vi "Teleop.vi"(10 "Match Info":T1={"Autonomous Elapsed Seconds"=0.0, "TeleOp Elapsed Seconds"=0.0, "Disabled Elapsed Seconds"=0.0, "Visited Autonomous"=FALSE, "Visited TeleOp"=FALSE, "Visited Disabled"=FALSE, "Autonomous Settings"={"Autonomous Style"=enum."Independent", "VI Refnum"=refnum}}, 11 "Call Context":T2) -> ()   [LabVIEW 2019]
doc: "This VI is called for each enabled TeleOp packet received from the DS. It is typically used to read from joysticks and other inputs and update I/O or setpoints for timed control loops. It should complete and return within 20 milliseconds or risk missing DS packets."
uses:
  <vilib>/Rock Robotics/WPI/DriverStation/WPI_DriverStationDerivedRobotMode.ctl
  <vilib>/Rock Robotics/WPI/DriverStation/WPI_DriverStationMatch Info.ctl
  Framework/Robot Global Data.vi
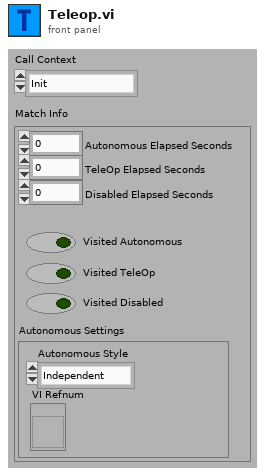
[diagram p1: front panel]
types:
  T1 = typedef "WPI_DriverStationMatch Info.ctl" = cluster{"Autonomous Elapsed Seconds":dbl, "TeleOp Elapsed Seconds":dbl, "Disabled Elapsed Seconds":dbl, "Visited Autonomous":bool, "Visited TeleOp":bool, "Visited Disabled":bool, "Autonomous Settings":cluster{"Autonomous Style":enum16{"Iterative", "Independent"}, "VI Refnum":refnum<vi>}}
  T2 = typedef "WPI_DriverStationDerivedRobotMode.ctl" = enum16{"Init", "Execute", "Stop"}
  T3 = typedef "Command Status Info.ctl" = cluster{"Name":string, "Status":T4, "notifier out":T5}
  T4 = typedef "Completion Status.ctl" = enum16{"Successful", "Aborted", "Incomplete"}
  T5 = typedef "Completion Notifier.ctl" = refnum<notifier>
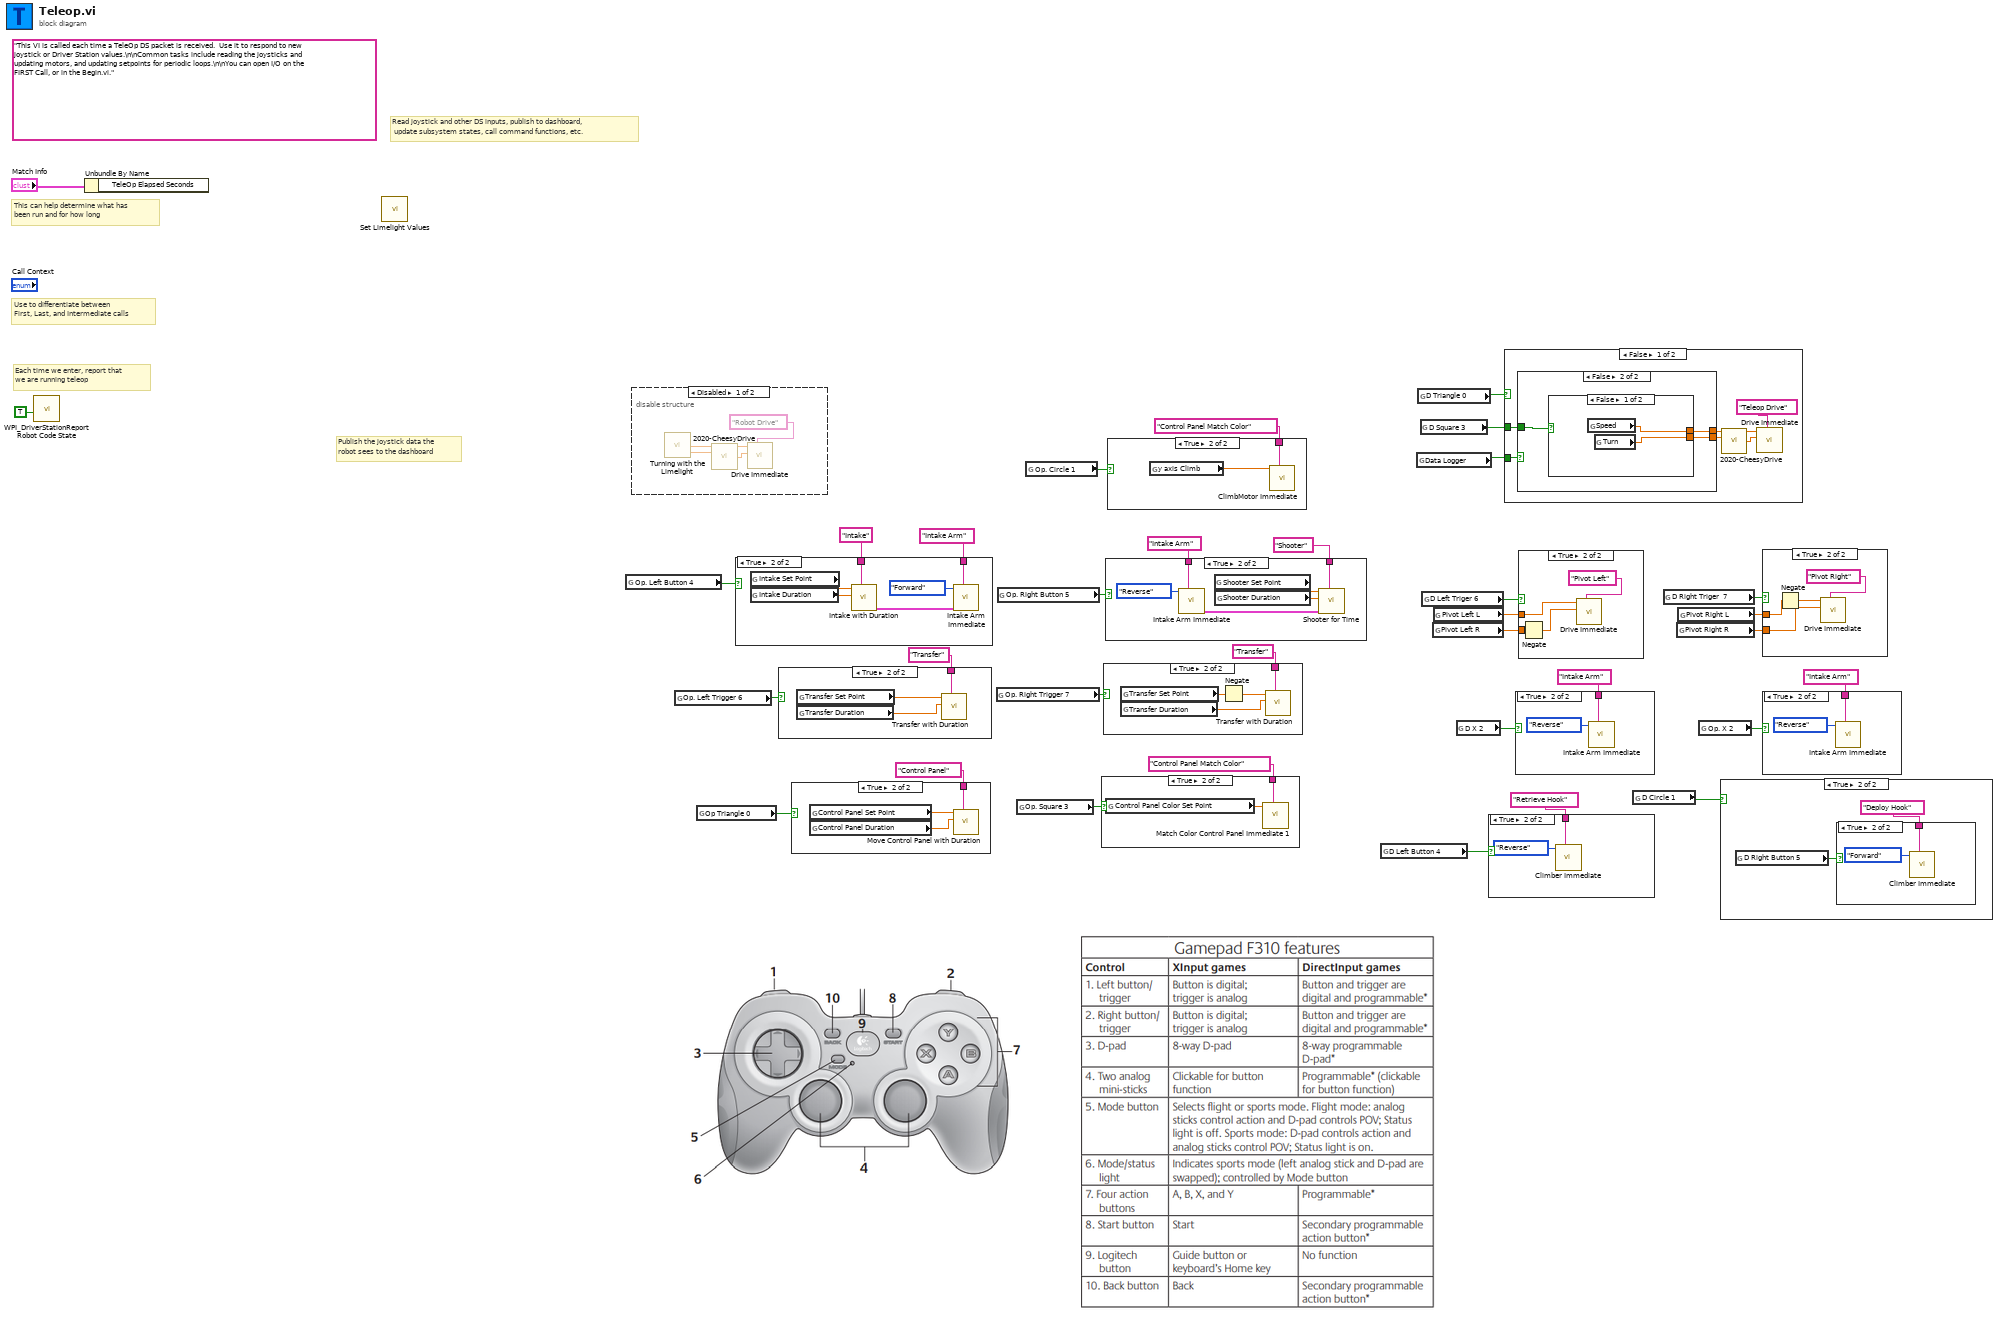
[diagram p0: block diagram]
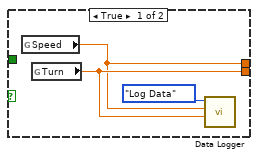
[diagram p8: hidden frame]
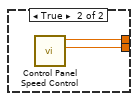
[diagram p9: hidden frame]
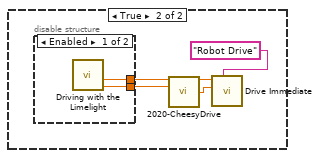
[diagram p10: hidden frame]
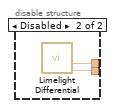
[diagram p11: hidden frame]
diagram:
  (unwired) "This VI is called each time a TeleOp DS packet is received.  Use it to respond to new joystick or Driver Station values.\n\nCommon tasks include reading the joysticks and updating motors, and updating setpoints for periodic loops.\n\nYou can open I/O on the FIRST Call, or in the Begin.vi."
  # "Publish the joystick data the\nrobot sees to the dashboard"
  # "Read joystick and other DS inputs, publish to dashboard,\n update subsystem states, call command functions, etc."
  # "Each time we enter, report that\nwe are running teleop"
  # "Use to differentiate between\nFirst, Last, and Intermediate calls"
  # "This can help determine what has\nbeen run and for how long"
  n1 = call <vilib>:"WPI_DriverStationReport Robot Code State.vi"("TeleOp"=TRUE ("Autonomous")) -> ()  [unwired: 10 in, 1 out]
  n2 = Unbundle By Name("Match Info") -> ()  [unwired: 1 out]
  n3 = call "Set Limelight Values.vi"() -> ()  [unwired: 12 in]
  n4 = global read "Robot Global Data.vi" "Op. Left Button 4"() -> (w32:bool)
  n5 = disable-structure shown="Disabled" {
    frame Disabled {
      n6 = call "Turning with the Limelight.vi"() -> ("TurnCommand"=w38:dbl, "Speed Command"=w39:dbl)  [unwired: 9 in, 1 out]
      n7 = call "2020-CheesyDrive.vi"("Throttle"=w39, "Wheel"=w38) -> ("Left PWM"=w37:dbl, "Right PWM"=w36:dbl)  [unwired: 12 in]
      n8 = call "Drive Immediate.vi"("Description"="Robot Drive", "Right Setpoint"=w36, "Left Setpoint"=w37) -> ()  [unwired: 8 in, 1 out]
    }
    frame Enabled {
    }
  }
  n9 = global read "Robot Global Data.vi" "Op. Left Trigger 6"() -> (w26:bool)
  n10 = global read "Robot Global Data.vi" "Op Triangle 0"() -> (w19:bool)
  n11 = case shown="True" w32 {
    tunnel: "Intake" ("refnum name") -> [_ w45]
    tunnel: "Intake Arm" ("refnum name") -> [_ w41]
    frame False {
    }
    frame True {
      n12 = global read "Robot Global Data.vi" "Intake Set Point"() -> (w44:dbl)
      n13 = global read "Robot Global Data.vi" "Intake Duration"() -> (w43:dbl)
      n14 = call "Intake with Duration.vi"("Description"=w45, "Duration (s)"=w43, "Setpoint"=w44) -> ("Command Info Out"=w40:T3)  [unwired: 8 in]
      n15 = call "Intake Arm Immediate.vi"("Description"=w41, "Command Info In"=w40, "Relay Value"=enum16{"Off", "On", "Forward", "Reverse"}."Forward") -> ()  [unwired: 8 in, 1 out]
    }
  }
  n16 = case shown="True" w26 {
    tunnel: "Transfer" ("refnum name") -> [_ w48]
    frame False {
    }
    frame True {
      n17 = global read "Robot Global Data.vi" "Transfer Set Point"() -> (w47:dbl)
      n18 = global read "Robot Global Data.vi" "Transfer Duration"() -> (w46:dbl)
      n19 = call "Transfer with Duration.vi"("Description"=w48, "Duration (s)"=w46, "Setpoint"=w47) -> ()  [unwired: 8 in, 1 out]
    }
  }
  n20 = case shown="True" w19 {
    tunnel: "Control Panel" ("refnum name") -> [_ w51]
    frame False {
    }
    frame True {
      n21 = global read "Robot Global Data.vi" "Control Panel Set Point"() -> (w50:dbl)
      n22 = global read "Robot Global Data.vi" "Control Panel Duration"() -> (w49:dbl)
      n23 = call "Move Control Panel with Duration.vi"("Description"=w51, "Duration (s)"=w49, "Setpoint"=w50) -> ()  [unwired: 8 in, 1 out]
    }
  }
  n24 = global read "Robot Global Data.vi" "Op. Right Trigger 7"() -> (w27:bool)
  n25 = global read "Robot Global Data.vi" "Op. Right Button 5"() -> (w28:bool)
  n26 = global read "Robot Global Data.vi" "Op. Square 3"() -> (w16:bool)
  n27 = global read "Robot Global Data.vi" "Op. Circle 1"() -> (w4:bool)
  n28 = case shown="True" w16 {
    tunnel: "Control Panel Match Color" ("refnum name") -> [_ w53]
    frame False {
    }
    frame True {
      n29 = global read "Robot Global Data.vi" "Control Panel Color Set Point"() -> (w52:dbl)
      n30 = call "Match Color Control Panel Immediate 1.vi"("Description"=w53, "Setpoint"=w52) -> ()  [unwired: 9 in, 1 out]
    }
  }
  n31 = case shown="True" w27 {
    tunnel: "Transfer" ("refnum name") -> [_ w57]
    frame False {
    }
    frame True {
      n32 = global read "Robot Global Data.vi" "Transfer Set Point"() -> (w55:dbl)
      n33 = global read "Robot Global Data.vi" "Transfer Duration"() -> (w54:dbl)
      n34 = Negate(x=w55) -> (-x=w56:dbl)
      n35 = call "Transfer with Duration.vi"("Description"=w57, "Duration (s)"=w54, "Setpoint"=w56) -> ()  [unwired: 8 in, 1 out]
    }
  }
  n36 = case shown="True" w28 {
    tunnel: "Shooter" ("refnum name") -> [_ w63]
    tunnel: "Intake Arm" ("refnum name") -> [_ w58]
    frame False {
    }
    frame True {
      n37 = call "Intake Arm Immediate.vi"("Description"=w58, "Relay Value"=enum16{"Off", "On", "Forward", "Reverse"}."Reverse") -> ("Command Info Out"=w59:T3)  [unwired: 9 in]
      n38 = global read "Robot Global Data.vi" "Shooter Set Point"() -> (w62:dbl)
      n39 = global read "Robot Global Data.vi" "Shooter Duration"() -> (w61:dbl)
      n40 = call "Shooter for Time.vi"("Description"=w63, "Command Info In"=w59, "Duration (s)"=w61, "Setpoint"=w62) -> ()  [unwired: 7 in, 1 out]
    }
  }
  n41 = case shown="True" w4 {
    tunnel: "Control Panel Match Color" ("refnum name") -> [_ w65]
    frame False {
    }
    frame True {
      n42 = global read "Robot Global Data.vi" "y axis Climb"() -> (w64:dbl)
      n43 = call "ClimbMotor Immediate.vi"("Description"=w65, "Setpoint"=w64) -> ()  [unwired: 9 in, 1 out]
    }
  }
  n44 = global read "Robot Global Data.vi" "D Left Button 4"() -> (w9:bool)
  n45 = global read "Robot Global Data.vi" "Data Logger"() -> (w2:bool)
  n46 = global read "Robot Global Data.vi" "D Triangle 0"() -> (w10:bool)
  n47 = global read "Robot Global Data.vi" "D Square 3"() -> (w1:bool)
  n48 = global read "Robot Global Data.vi" "D Left Triger 6"() -> (w24:bool)
  n49 = global read "Robot Global Data.vi" "Pivot Left R"() -> (w13:dbl)
  n50 = global read "Robot Global Data.vi" "Pivot Left L"() -> (w14:dbl)
  n51 = global read "Robot Global Data.vi" "D X 2"() -> (w17:bool)
  n52 = case shown="True" w9 {
    tunnel: "Retrieve Hook" ("refnum name") -> [_ w66]
    frame False {
    }
    frame True {
      n53 = call "Climber Immediate.vi"("Description"=w66, "Value"=enum16{"Off", "On", "Forward", "Reverse"}."Reverse" ("Relay Value")) -> ()  [unwired: 9 in, 1 out]
    }
  }
  n54 = case shown="False" w10 {
    tunnel: w2 -> [w69 _]
    tunnel: w1 -> [w68 _]
    frame False {
      n55 = case shown="False" w69 {
        tunnel: [w77 w80] -> w72
        tunnel: [w76 w79] -> w71
        tunnel: w68 -> [_ w78]
        frame True {
          n56 = global read "Robot Global Data.vi" "Speed"() -> (w76:dbl)
          n57 = global read "Robot Global Data.vi" "Turn"() -> (w77:dbl)
          n58 = call "Data Logger.vi"("Turn X joystick"=w77, "Speed Y Joystick"=w76, "Function"=enum16{"Start Log", "Log Data", "Stop Log"}."Log Data") -> ()  [unwired: 7 in, 2 out]
        }
        frame False {
          n59 = case shown="False" w78 {
            tunnel: [w82 w83] -> w80
            tunnel: [w81 w84] -> w79
            frame False {
              n60 = global read "Robot Global Data.vi" "Speed"() -> (w81:dbl)
              n61 = global read "Robot Global Data.vi" "Turn"() -> (w82:dbl)
            }
            frame True {
              n62 = call "Control Panel Speed Control.vi"() -> ("Turn"=w83:dbl, "Speed"=w84:dbl)  [unwired: 10 in]
            }
          }
        }
      }
      n63 = call "2020-CheesyDrive.vi"("Throttle"=w71, "Wheel"=w72) -> ("Left PWM"=w73:dbl, "Right PWM"=w74:dbl)  [unwired: 12 in]
      n64 = call "Drive Immediate.vi"("Description"="Teleop Drive", "Right Setpoint"=w74, "Left Setpoint"=w73) -> ()  [unwired: 8 in, 1 out]
    }
    frame True {
      n65 = disable-structure shown="Enabled" {
        disable-tunnel: [w91 w92] -> w85
        disable-tunnel: [w90 w93] -> w86
        frame Enabled {
          n66 = call "Driving with the Limelight.vi"() -> ("TurnCommand"=w91:dbl, "SpeedCommand"=w90:dbl)  [unwired: 9 in, 1 out]
        }
        frame Disabled {
          n67 = call "Limelight Differential.vi"() -> ("DriveCommand"=w92:dbl, "SteerCommand"=w93:dbl)  [unwired: 9 in, 1 out]
        }
      }
      n68 = call "2020-CheesyDrive.vi"("Throttle"=w86, "Wheel"=w85) -> ("Left PWM"=w88:dbl, "Right PWM"=w89:dbl)  [unwired: 12 in]
      n69 = call "Drive Immediate.vi"("Description"="Robot Drive", "Right Setpoint"=w89, "Left Setpoint"=w88) -> ()  [unwired: 8 in, 1 out]
    }
  }
  n70 = case shown="True" w17 {
    tunnel: "Intake Arm" ("refnum name") -> [_ w94]
    frame False {
    }
    frame True {
      n71 = call "Intake Arm Immediate.vi"("Description"=w94, "Relay Value"=enum16{"Off", "On", "Forward", "Reverse"}."Reverse") -> ()  [unwired: 9 in, 1 out]
    }
  }
  n72 = case shown="True" w24 {
    tunnel: w14 -> [_ w98]
    tunnel: w13 -> [_ w97]
    frame False {
    }
    frame True {
      n73 = Negate(x=w97) -> (-x=w96:dbl)
      n74 = call "Drive Immediate.vi"("Description"="Pivot Left", "Right Setpoint"=w96, "Left Setpoint"=w98) -> ()  [unwired: 8 in, 1 out]
    }
  }
  n75 = global read "Robot Global Data.vi" "D Circle 1"() -> (w3:bool)
  n76 = global read "Robot Global Data.vi" "D Right Triger  7"() -> (w23:bool)
  n77 = global read "Robot Global Data.vi" "Pivot Right R"() -> (w11:dbl)
  n78 = global read "Robot Global Data.vi" "Pivot Right L"() -> (w12:dbl)
  n79 = global read "Robot Global Data.vi" "Op. X 2"() -> (w7:bool)
  n80 = case shown="True" w3 {
    frame False {
    }
    frame True {
      n81 = global read "Robot Global Data.vi" "D Right Button 5"() -> (w100:bool)
      n82 = case shown="True" w100 {
        tunnel: "Deploy Hook" ("refnum name") -> [_ w102]
        frame False {
        }
        frame True {
          n83 = call "Climber Immediate.vi"("Description"=w102, "Value"=enum16{"Off", "On", "Forward", "Reverse"}."Forward" ("Relay Value")) -> ()  [unwired: 9 in, 1 out]
        }
      }
    }
  }
  n84 = case shown="True" w23 {
    tunnel: w12 -> [_ w106]
    tunnel: w11 -> [_ w105]
    frame False {
    }
    frame True {
      n85 = Negate(x=w106) -> (-x=w104:dbl)
      n86 = call "Drive Immediate.vi"("Description"="Pivot Right", "Right Setpoint"=w105, "Left Setpoint"=w104) -> ()  [unwired: 8 in, 1 out]
    }
  }
  n87 = case shown="True" w7 {
    tunnel: "Intake Arm" ("refnum name") -> [_ w108]
    frame False {
    }
    frame True {
      n88 = call "Intake Arm Immediate.vi"("Description"=w108, "Relay Value"=enum16{"Off", "On", "Forward", "Reverse"}."Reverse") -> ()  [unwired: 9 in, 1 out]
    }
  }
